vi "read_power.vi"() -> (0 "Power (%)":dbl)   [LabVIEW 2011]
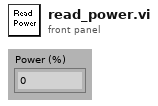
[diagram p1: front panel]
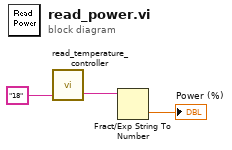
[diagram p0: block diagram]
diagram:
  n1 = call "read_temperature_controller.vi"("Command"="18") -> ("Value"=w2:string)  [unwired: 2 in, 1 out]
  n2 = Fract/Exp String To Number(string=w2) -> (number=→"Power (%)":dbl)  [unwired: 4 out]
